vi "System@AddExternalDevice__Parameter.vi"(1 "ParamterIn":string) -> (0 "ParamterOut":string)   [LabVIEW 2019]
panel:
  in  "Parameter":string(combo)
  in  "Driver":string(combo)
  in  "Device":string(combo)
  in  "Confirm":bool
  # "System@AddExternalDevice $Device,$Driver,$Parameter"
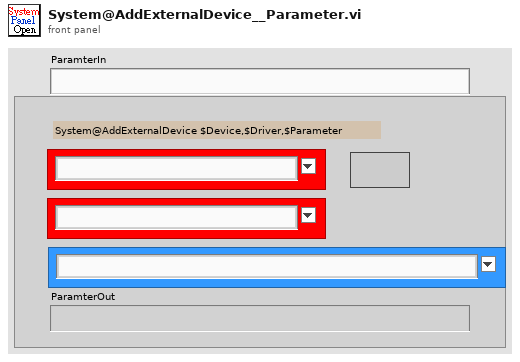
[diagram p1: front panel]
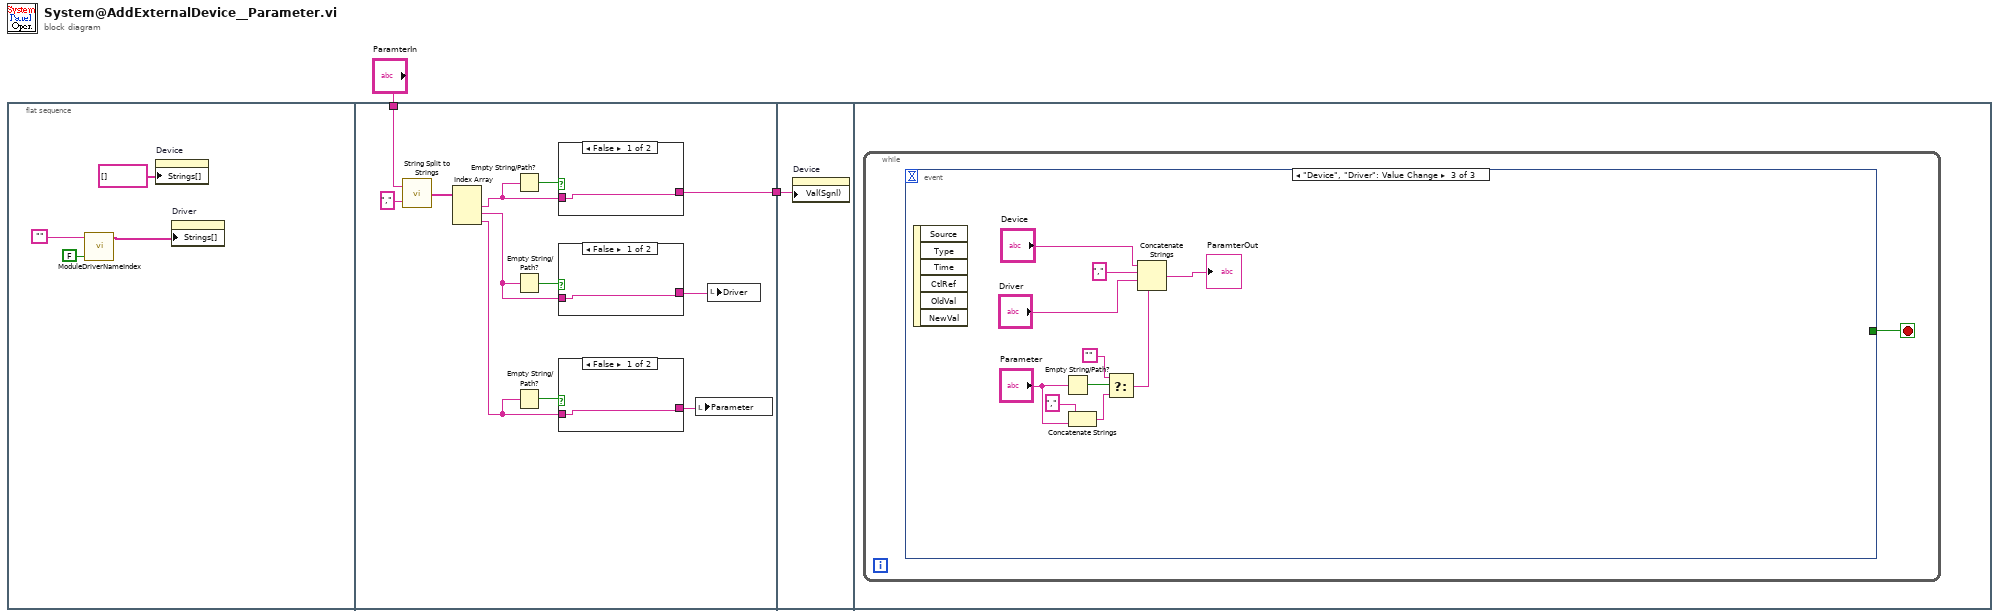
[diagram p0: block diagram]
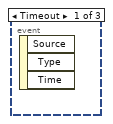
[diagram p5: hidden frame]
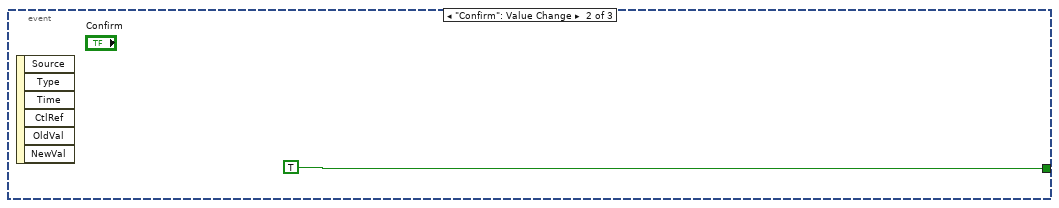
[diagram p6: hidden frame]
diagram:
  n1 = flat-sequence {
    tunnel: "ParamterIn" -> [w14]
    tunnel: [w17] -> w1
    tunnel: w1 -> [w25]
    frame #0 {
      n2 = call "ModuleDriverNameIndex.vi"("Init"=FALSE, "DriverName"="") -> ("DriverNameList"=w4:string[])  [unwired: 1 in, 2 out]
      n3 = property on="Device" class="CmbBox"("Strings[]"=string[] [] ("Strings []")) -> ()  [unwired: 2 in, 2 out]
      n4 = property on="Driver" class="CmbBox"("Strings[]"=w4) -> ()  [unwired: 2 in, 2 out]
    }
    frame #1 {
      n5 = call "String Split to Strings.vi"("search string/char (-)"=",", "String"=w14) -> ("Array"=w12:string[])
      n6 = Index Array(array=w12) -> (element #1=w11:string, element #2=w10:string, element #3=w8:string)  [unwired: 3 in]
      n7 = Empty String/Path?(string/path=w11) -> (empty?=w18:bool)
      n8 = Empty String/Path?(string/path=w10) -> (empty?=w16:bool)
      n9 = Empty String/Path?(string/path=w8) -> (empty?=w9:bool)
      n10 = case shown="False" w18 {
        tunnel: w11 -> [w23 w24]
        tunnel: [w23 w24] -> w17
        frame False {
        }
        frame True {
        }
      }
      n11 = case shown="False" w16 {
        tunnel: w10 -> [w21 w22]
        tunnel: [w21 w22] -> w15
        frame False {
        }
        frame True {
        }
      }
      n12 = case shown="False" w9 {
        tunnel: w8 -> [w19 w20]
        tunnel: [w19 w20] -> w7
        frame False {
        }
        frame True {
        }
      }
      n13 = local write "Parameter"(w7) -> ()
      n14 = local write "Driver"(w15) -> ()
    }
    frame #2 {
      n15 = property on="Device" class="CmbBox"("Val(Sgnl)"=w25) -> ()  [unwired: 2 in, 2 out]
    }
    frame #3 {
      n16 = while {
        stop <- w26 stop-if-true
        n17 = event shown="[2] \"Device\", \"Driver\": Value Change" {
          selector: _ -> [_ _ _]
          dyn-events: _ -> [_ _ _]
          timeout: _ -> [_ _ _]
          tunnel: [_ TRUE _] -> w26
          event Timeout {
            n18 = event-data() -> ()  [unwired: 1 in, 3 out]
          }
          event "Confirm": Value Change {
            n19 = event-data() -> ()  [unwired: 1 in, 6 out]
          }
          event "Device", "Driver": Value Change {
            n20 = event-data() -> ()  [unwired: 1 in, 6 out]
            n21 = Empty String/Path?(string/path="Parameter") -> (empty?=w34:bool)
            n22 = Concatenate Strings("," ("search string/char (-)"), "Parameter") -> (w31:string)
            n23 = Select(t="", s=w34, f=w31) -> (s? t:f=w28:string)
            n24 = Concatenate Strings("Device", "," ("string"), "Driver", w28) -> (→"ParamterOut":string)
          }
        }
      }
    }
  }
